vi "NI VeriStand - Get Custom Device Channel Data.vi"(8 "error in (no error)":errorcluster, 11 "Channel Ref in":T3 format="%.0x") -> (0 "error out":errorcluster, 1 "Channel":T1, 2 "Channel Name":string, 3 "Channel Ref out":T3 format="%.0x", 4 "Found":bool, 5 "GUID":string)   [LabVIEW 2020, in "Custom Device API.lvlib"]
doc: "Returns information about the channel specified by <B>Channel Ref in</B>."
uses:
  <vilib>/NI VeriStand/Custom Device API/Custom Device API.lvlib
  <vilib>/NI VeriStand/Custom Device API/Custom Device Item Ref.ctl
  <vilib>/NI VeriStand/Custom Device API/Custom Device Channel.ctl
  <vilib>/NI VeriStand/Custom Device API/Custom Device Channel Type.ctl
  7fa9cd82-b288-493d-b437-9924279ebaf6.vi
  <vilib>/NI VeriStand/Custom Device API/Custom Device Offline Path.vi
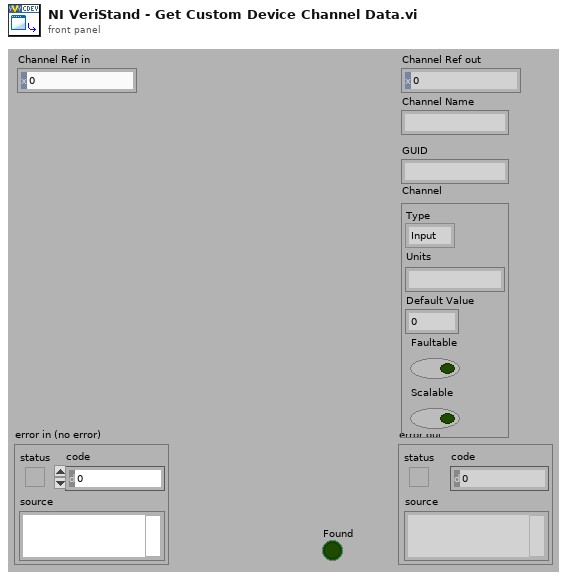
[diagram p1: front panel]
types:
  T1 = typedef "Custom Device API.lvlib/Custom Device Channel.ctl" = cluster{"Type":T2, "Units":string, "Default Value":dbl, "Faultable":bool, "Scalable":bool}
  T2 = typedef "Custom Device API.lvlib/Custom Device Channel Type.ctl" = enum16{"Input", "Output"}
  T3 = typedef "Custom Device API.lvlib/Custom Device Item Ref.ctl" = u64
  T4 = typedef "Custom Devices Storage.lvlib/Custom Device Channel.ctl" = cluster{"Type":T5, "Units":string, "Default Value":dbl, "Faultable":bool, "Scalable":bool}
  T5 = typedef "Custom Devices Storage.lvlib/Custom Device Channel Type.ctl" = enum16{"Input", "Output"}
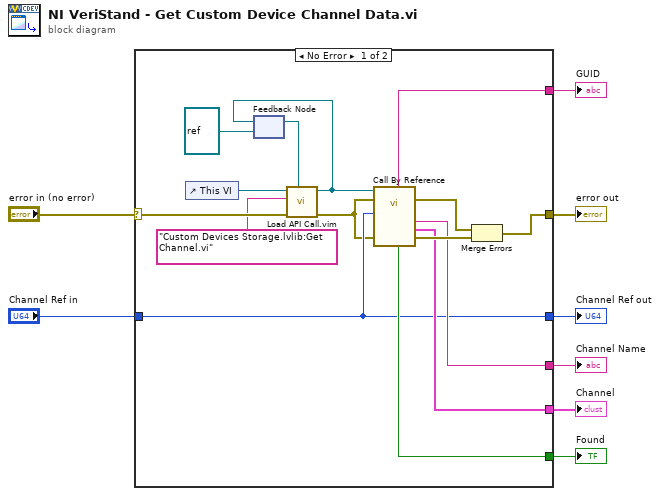
[diagram p0: block diagram]
diagram:
  n1 = case shown="No Error" "error in (no error)" {
    selector: "error in (no error)" -> [w14 w25]
    tunnel: "Channel Ref in" -> [w17 w24]
    tunnel: [w17 w24] -> w7
    tunnel: [w22 _] -> w6
    tunnel: [w21 _] -> w5
    tunnel: [w20 w25] -> w4
    tunnel: [w19 _] -> w3
    tunnel: [w18 _] -> w2
    frame No Error {
      n2 = control-ref of="This VI"() -> (w15:refnum<vi>)
      n3 = feedback #1(refnum<vi> refnum ("type specifier VI Refnum (for type only)")) -> (w16:refnum<vi>)
      n4 = call "Load API Call.vim"("VI reference in"=w16, "error in (no error)"=w14, "VI qualified name"="Custom Devices Storage.lvlib:Get Channel.vi", "Caller VI ref"=w15) -> ("error out"=w13:errorcluster, "VI reference"=w12:refnum<vi>)  [unwired: 6 in]
      n5 = feedback-in #1(w12) -> ()
      n6 = call-by-ref "?"(reference=w12, error in=w13, 8:"error in (no error)"=w13, "Channel Ref in"=w17) -> (error out=w9:errorcluster, 0:"error out"=w23:errorcluster, "Channel"=w19:T4, "Channel Name"=w22:string, "Found"=w21:bool, "GUID"=w18:string)  [unwired: 4 in, 2 out]
      n7 = Merge Errors(w9, w23) -> (w20:errorcluster)
    }
    frame Error {
    }
  }
  "Channel Ref out" <- w7
  "error out" <- w4
  "Channel" <- w3
  "Found" <- w5
  "GUID" <- w2
  "Channel Name" <- w6
